vi "GOMDBTS2048 calib Az Set Calib Lamp.vi"(8 "error in (no error)":errorcluster, 9 "name":string, 10 "values":dbl[](array[numeric]), 11 "handle":i32) -> (0 "error out":errorcluster, 3 "function return":i32)   [LabVIEW 2015, in "GOMDBTS2048.lvlib"]
doc: "GOBTS2048DLL int __stdcall GOMDBTS2048_calibTristimulusSetXYZ(int handle, double* valuesX, double* valuesY, double* valuesZ); GOBTS2048DLL int __stdcall GOMDBTS2048_calibTristimulusGetXYZ(int handle, double* valuesX, double* valuesY, double* valuesZ); GOBTS2048DLL int __stdcall GOMDBTS2048_calibAzSetCalibLamp(int handle, double* values, char* name);"
uses:
  GOMDBTS2048.lvlib
  runtime/GOMDBTS2048.dll
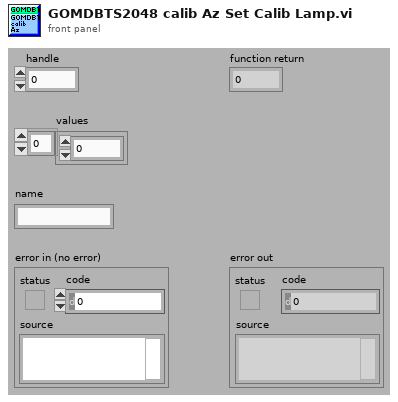
[diagram p1: front panel]
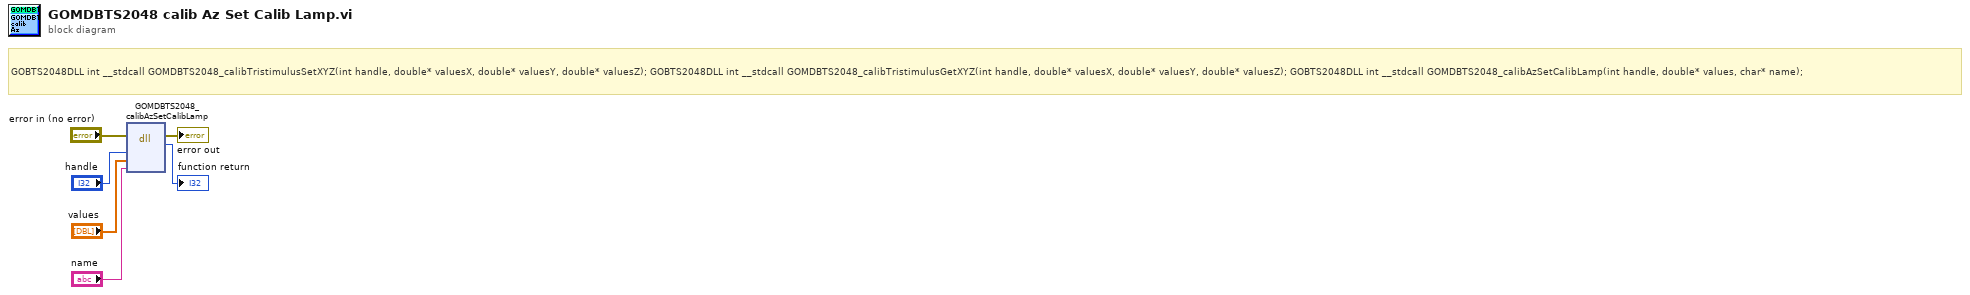
[diagram p0: block diagram]
diagram:
  # "GOBTS2048DLL int __stdcall GOMDBTS2048_calibTristimulusSetXYZ(int handle, double* valuesX, double* valuesY, double* valuesZ); GOBTS2048DLL int __stdcall GOMDBTS2048_calibTristimulusGetXYZ(int handle, double* valuesX, double* valuesY, double* valuesZ); GOBTS2048DLL int __stdcall GOMDBTS2048_calibAzSetCalibLamp(int handle, double* values, char* name);"
  n1 = dll-call lib="C:/Users/rkoch/Documents/GO_Library/runtime/GOMDBTS2048.*" fn="GOMDBTS2048_calibAzSetCalibLamp"(error in="error in (no error)", "handle"="handle", "values"="values", "name"="name") -> (error out=→"error out":errorcluster, →"function return":i32)  [unwired: 5 in, 1 out]
